vi "Image Display Mouse Wheel Zoom.vi"(8 "Error In":errorcluster, 10 "Mouse Wheel Delta":i32, 11 "Image Control Refnum":T1) -> (0 "Error Out":errorcluster)   [LabVIEW 2021, in "Image.lvlib"]
uses:
  Image.lvlib
  Image Control Refnum.ctl
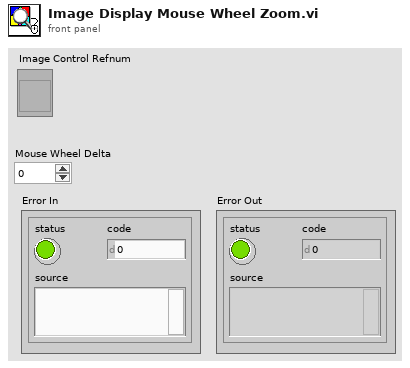
[diagram p1: front panel]
types:
  T1 = typedef "Image.lvlib/Image Control Refnum.ctl" = refnum<vi>
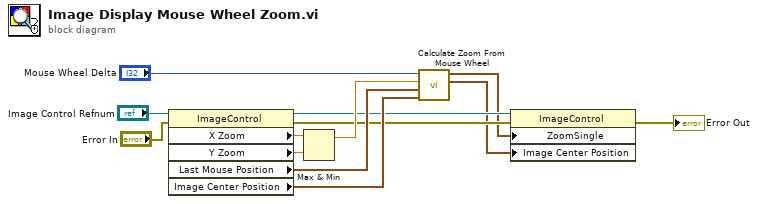
[diagram p0: block diagram]
diagram:
  n1 = property class="ImageControl"(reference="Image Control Refnum", error in="Error In") -> (reference out=w5:T1, error out=w4:errorcluster, "X Zoom"=w10:sgl, "Y Zoom"=w9:sgl, "Last Mouse Position"=w7:cluster{"X":i32, "Y":i32}, "Image Center Position"=w6:cluster{"X":u32, "Y":u32})
  n2 = Max & Min(x=w10, y=w9) -> (max(x,y)=w8:sgl)  [unwired: 1 out]
  n3 = call "Calculate Zoom From Mouse Wheel.vi"("Image Center Position"=w6, "Last Mouse Position"=w7, "Current Zoom Factor"=w8, "Delta"="Mouse Wheel Delta") -> ("New Center Position"=w2:cluster{dbl, dbl}, "New Zoom"=w3:cluster{dbl, dbl})  [unwired: 6 in]
  n4 = property class="ImageControl"(reference=w5, error in=w4, "ZoomSingle"=w3, "Image Center Position"=w2) -> (error out=→"Error Out":errorcluster)  [unwired: 1 out]
